vi "LockinDAQ.setSweep.vi"(8 "error in (no error)":errorcluster, 10 "setSweep":T1 {"Sweep IV Step (V)" format="%#_6p"; "Sweep End (V)" format="%#_6p"; "Sweep Start (V)" format="%#_6p"; "Sweep Lockin Time (s)" format="%#_6p"}, 11 "LockinDAQ":refnum<class "LockinDAQ.lvclass">) -> (0 "error out":errorcluster, 3 "LockinDAQ out":refnum<class "LockinDAQ.lvclass">)   [LabVIEW 2016, in "LockinDAQ.lvclass"]
doc: "---------------------------------------------------------------\nJKI State Machine Objects™\nhttp://jki.net/state-machine-objects/\nCopyright (C) 2005-2015, JKI <info@jki.net>\nALL RIGHTS RESERVEDJKI State Machine Objects (SMO) 1.0.0.4\nJKI - JKI\nCopyright (c) 2015, JKI"
uses:
  LockinDAQ.lvclass
  Typedefs/Sweep Configuration--Cluster.ctl
  LockinDAQ.lvclass/LockinDAQ.ctl
panel:
  # "For instructions on how to use the JKI State Machine Objects, examples and video tutorials, visit:\nhttp://jki.net/state-machine-objects/\n\nJKI State Machine Objects™\nhttp://jki.net/state-machine-objects/\nCopyright (C) 2005-2015, JKI <info@jki.net>\nALL RIGHTS RESERVED"
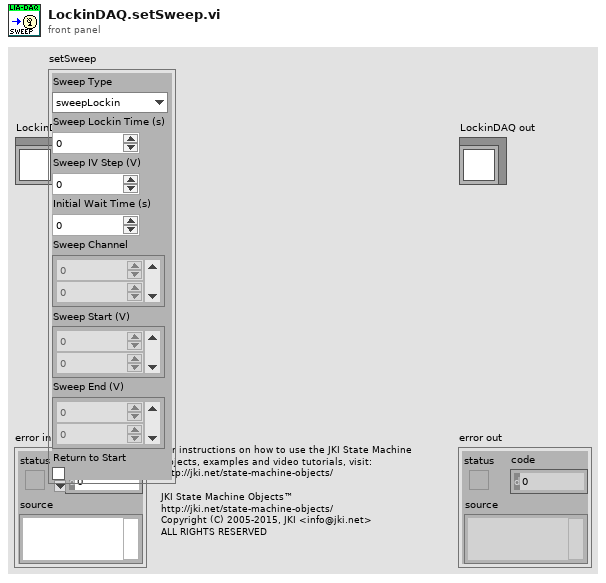
[diagram p1: front panel]
types:
  T1 = typedef "LockinDAQ.lvclass/Sweep Configuration--Cluster.ctl" = cluster{"Sweep Type":enum16{"sweepLockin", "sweepIV"}, "Sweep Lockin Time (s)":dbl, "Sweep IV Step (V)":dbl, "Initial Wait Time (s)":dbl, "Sweep Channel":i32[], "Sweep Start (V)":dbl[], "Sweep End (V)":dbl[], "Return to Start":bool}
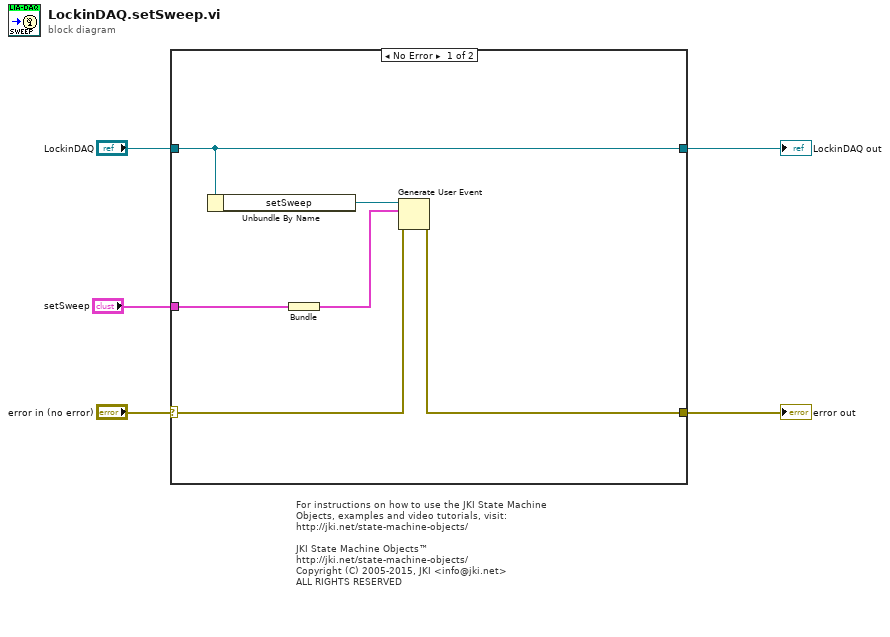
[diagram p0: block diagram]
diagram:
  # "For instructions on how to use the JKI State Machine Objects, examples and video tutorials, visit:\nhttp://jki.net/state-machine-objects/\n\nJKI State Machine Objects™\nhttp://jki.net/state-machine-objects/\nCopyright (C) 2005-2015, JKI <info@jki.net>\nALL RIGHTS RESERVED"
  n1 = case shown="No Error" "error in (no error)" {
    selector: "error in (no error)" -> [w11 w13]
    tunnel: [w9 w13] -> w4
    tunnel: [w8 w12] -> w5
    tunnel: "LockinDAQ" -> [w8 w12]
    tunnel: "setSweep" -> [w6 _]
    frame No Error {
      n2 = Unbundle By Name(w8) -> ("setSweep"=w10:refnum<user-event>)
      n3 = Bundle("setSweep"=w6) -> (w7:cluster{"setSweep":T1})  [unwired: 1 in]
      n4 = Generate User Event(user event=w10, event data cluster=w7, error in=w11) -> (error out=w9:errorcluster)  [unwired: 1 in, 1 out]
    }
    frame Error {
    }
  }
  "error out" <- w4
  "LockinDAQ out" <- w5
